vi "UTL_Read_Write Controllers.vi"(8 "error in":errorcluster) -> (0 "error out":errorcluster, 2 "StatusCtrl":T1(array[cluster]), 5 "Results":dbl[][][](array[numeric]))   [LabVIEW 2024]
uses:
  <vilib>/Plasmionique/MB Master/MB_Master_Serial/MB_Master_Serial.lvclass
  Variable global de carga.vi
  <vilib>/Plasmionique/MB Master/MB Master.lvlib
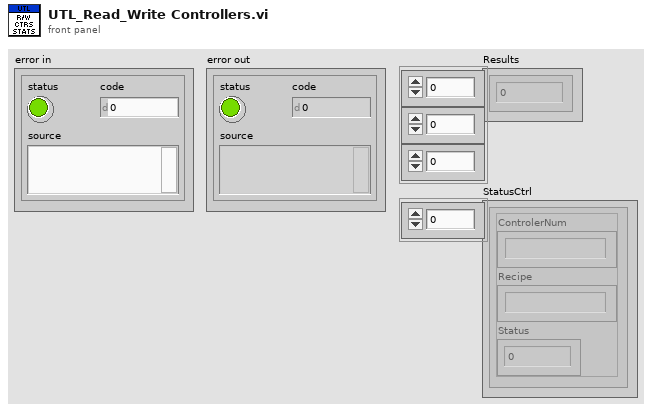
[diagram p1: front panel]
types:
  T1 = cluster{"ControlerNum":string, "Recipe":string, "Status":u32}[]
  T2 = typedef "Control 2.ctl" = refnum<class "MB_Master_Serial.lvclass">[]
  T3 = cluster{"ControlerNum":string, "Recipe":string, "Status":u32}
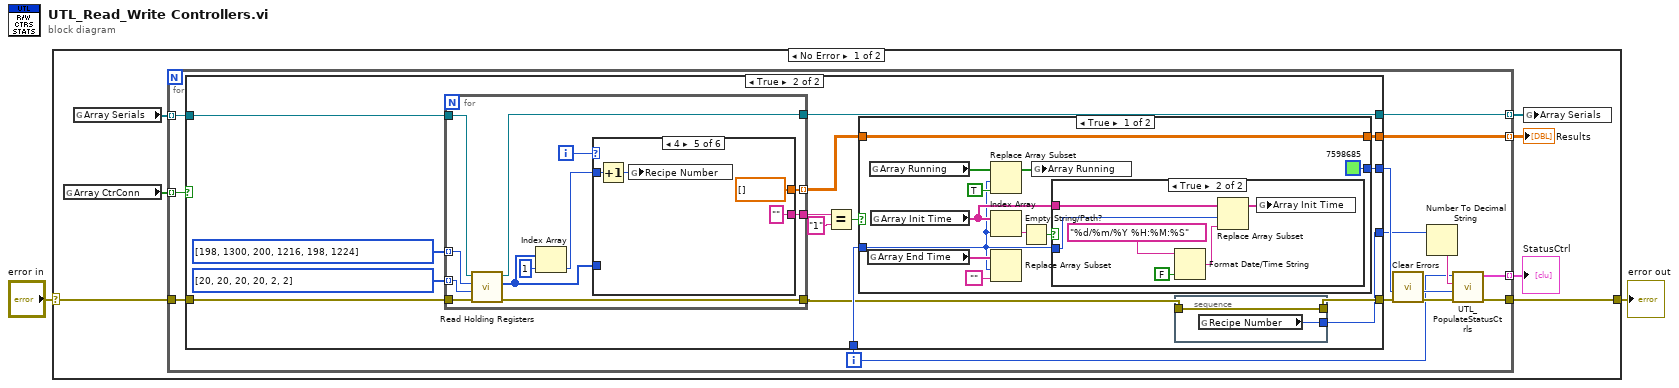
[diagram p0: block diagram]
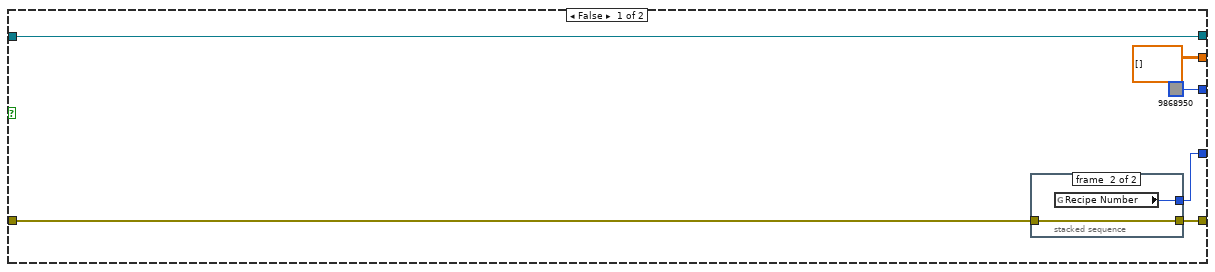
[diagram p2: hidden frame]
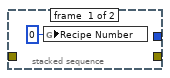
[diagram p3: hidden frame]
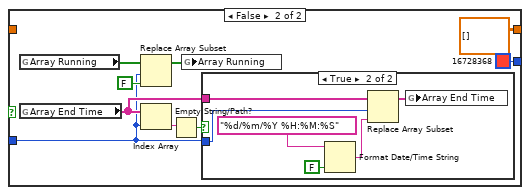
[diagram p5: hidden frame]
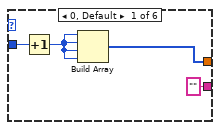
[diagram p7: hidden frame]
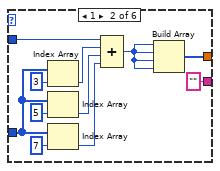
[diagram p8: hidden frame]
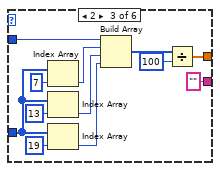
[diagram p9: hidden frame]
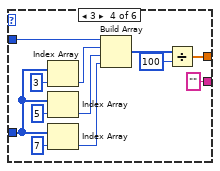
[diagram p10: hidden frame]
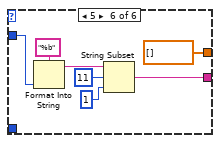
[diagram p11: hidden frame]
diagram:
  n1 = case shown="No Error" "error in" {
    selector: "error in" -> [w8 w143]
    tunnel: [w9 w143] -> w1
    frame No Error {
      n2 = global read "Variable global de carga.vi" "Array CtrConn"() -> (w3:bool[])
      n3 = global read "Variable global de carga.vi" "Array Serials"() -> (w7:T2)
      n4 = for {
        tunnel: w7 -> [w21] mode=indexing
        tunnel: [w20] -> w6 mode=indexing
        tunnel: [w19] -> w5 mode=indexing
        tunnel: w8 -> [w22]
        tunnel: [w18] -> w9
        tunnel: [w17] -> w4 mode=indexing
        tunnel: w3 -> [w11] mode=indexing
        i -> [w12]
        n5 = case shown="True" w11 {
          tunnel: w22 -> [w23 w46]
          tunnel: w21 -> [w28 w41]
          tunnel: [w28 w40] -> w20
          tunnel: [dbl[][] [] w37] -> w19
          tunnel: w12 -> [_ w36]
          tunnel: [w24 w33] -> w14
          tunnel: [u32 9868950 ("Status") w35] -> w13
          tunnel: [w25 w32] -> w10
          frame False {
            n6 = stacked-sequence {
              tunnel: [_ w31] -> w25
              tunnel: [_ w30] -> w24
              tunnel: w23 -> [_ w30]
              frame #0 {
                n7 = global write "Variable global de carga.vi" "Recipe Number"(u16 0 ("Recipe Number")) -> ()
              }
              frame #1 {
                n8 = global read "Variable global de carga.vi" "Recipe Number"() -> (w31:u16)
              }
            }
          }
          frame True {
            n9 = for {
              tunnel: i32[] [198, 1300, 200, 1216, 198, 1224] -> [w88] mode=indexing
              tunnel: [w91] -> w40
              tunnel: [w92] -> w34
              tunnel: [w89] -> w38 mode=indexing
              tunnel: i32[] [20, 20, 20, 20, 2, 2] -> [w87] mode=indexing
              tunnel: w46 -> [w83]
              tunnel: w41 -> [w82]
              tunnel: [w81] -> w42
              i -> [w90]
              n10 = call <vilib>:"Read Holding Registers.vi"("error in (no error)"=w83, "quantity"=w87, "starting address"=w88, "MB session in"=w82) -> ("error out"=w92:errorcluster, "Registers"=w84:u16[], "MB session out"=w91:refnum<class "MB_Master_Serial.lvclass">)  [unwired: 5 in]
              n11 = Index Array(array=w84, index=1) -> (element=w85:u16)
              n12 = case shown="4" w90 {
                tunnel: w84 -> [_ w104 w116 w128 _ _]
                tunnel: [w95 w99 w110 w122 dbl[] [] dbl[] []] -> w89
                tunnel: w85 -> [w94 w98 w109 w121 w135 w138]
                tunnel: ["" "" "" "" "" w136] -> w81
                frame 0, Default {
                  n13 = Increment(x=w94) -> (x+1=w96:u16)
                  n14 = Build Array(w96, w96, w96, w96) -> (w95:u16[])
                }
                frame 1 {
                  n15 = Index Array(array=w104, index=3) -> (element=w103:u16)
                  n16 = Index Array(array=w104, index=5) -> (element=w102:u16)
                  n17 = Index Array(array=w104, index=7) -> (element=w101:u16)
                  n18 = Compound Arithmetic op=ADD(w98, w103, w102, w101) -> (w100:u16)
                  n19 = Build Array(w100, w100, w100, w100) -> (w99:u16[])
                }
                frame 2 {
                  n20 = Index Array(array=w116, index=7) -> (element=w115:u16)
                  n21 = Index Array(array=w116, index=13) -> (element=w114:u16)
                  n22 = Index Array(array=w116, index=19) -> (element=w113:u16)
                  n23 = Build Array(w109, w115, w114, w113) -> (w111:u16[])
                  n24 = Divide(x=w111, y=100) -> (x/y=w110:dbl[])
                }
                frame 3 {
                  n25 = Index Array(array=w128, index=3) -> (element=w127:u16)
                  n26 = Index Array(array=w128, index=5) -> (element=w126:u16)
                  n27 = Index Array(array=w128, index=7) -> (element=w125:u16)
                  n28 = Build Array(w121, w127, w126, w125) -> (w123:u16[])
                  n29 = Divide(x=w123, y=100) -> (x/y=w122:dbl[])
                }
                frame 4 {
                  n30 = Increment(x=w135) -> (x+1=w132:u16)
                  n31 = global write "Variable global de carga.vi" "Recipe Number"(w132) -> ()
                }
                frame 5 {
                  n32 = Format Into String(format string="%b", w138) -> (resulting string=w142:string)  [unwired: 2 in, 1 out]
                  n33 = String Subset(string=w142, offset (0)=11, length (rest)=1 ("length (rest)")) -> (substring=w136:string)
                }
              }
            }
            n34 = Equal?(x=w42, y="1") -> (x = y?=w39:bool)
            n35 = case shown="True" w39 {
              tunnel: w36 -> [w51 w68]
              tunnel: w38 -> [w50 _]
              tunnel: [w50 dbl[][] []] -> w37
              tunnel: [u32 7598685 ("Status 3") u32 16728368 ("Status 4")] -> w35
              frame True {
                n36 = global read "Variable global de carga.vi" "Array End Time"() -> (w53:string[])
                n37 = global read "Variable global de carga.vi" "Array Running"() -> (w55:bool[])
                n38 = global read "Variable global de carga.vi" "Array Init Time"() -> (w57:string[])
                n39 = Replace Array Subset(array=w55, new element=TRUE, index=w51) -> (w54:bool[])
                n40 = Index Array(array=w57, index=w51) -> (element=w59:string)
                n41 = Replace Array Subset(array=w53, new element="" ("new element/subarray"), index=w51) -> ()  [unwired: 1 out]
                n42 = Empty String/Path?(string/path=w59) -> (empty?=w58:bool)
                n43 = global write "Variable global de carga.vi" "Array Running"(w54) -> ()
                n44 = case shown="True" w58 {
                  tunnel: w51 -> [_ w62]
                  tunnel: w57 -> [_ w63]
                  frame False {
                  }
                  frame True {
                    n45 = Format Date/Time String(time format string (%c)="%d/%m/%Y %H:%M:%S", UTC format=FALSE) -> (date/time string=w60:string)  [unwired: 1 in]
                    n46 = Replace Array Subset(array=w63, new element=w60, index=w62) -> (w61:string[])
                    n47 = global write "Variable global de carga.vi" "Array Init Time"(w61) -> ()
                  }
                }
              }
              frame False {
                n48 = global read "Variable global de carga.vi" "Array Running"() -> (w70:bool[])
                n49 = global read "Variable global de carga.vi" "Array End Time"() -> (w72:string[])
                n50 = Replace Array Subset(array=w70, new element=FALSE, index=w68) -> (w69:bool[])
                n51 = Index Array(array=w72, index=w68) -> (element=w74:string)
                n52 = Empty String/Path?(string/path=w74) -> (empty?=w73:bool)
                n53 = global write "Variable global de carga.vi" "Array Running"(w69) -> ()
                n54 = case shown="True" w73 {
                  tunnel: w68 -> [_ w77]
                  tunnel: w72 -> [_ w78]
                  frame False {
                  }
                  frame True {
                    n55 = Format Date/Time String(time format string (%c)="%d/%m/%Y %H:%M:%S", UTC format=FALSE) -> (date/time string=w75:string)  [unwired: 1 in]
                    n56 = Replace Array Subset(array=w78, new element=w75, index=w77) -> (w76:string[])
                    n57 = global write "Variable global de carga.vi" "Array End Time"(w76) -> ()
                  }
                }
              }
            }
            n58 = stacked-sequence {
              tunnel: [w48] -> w32
              tunnel: w34 -> [w47]
              tunnel: [w47] -> w33
              frame #0 {
                n59 = global read "Variable global de carga.vi" "Recipe Number"() -> (w48:u16)
              }
            }
          }
        }
        n60 = call <vilib>:"Clear Errors.vi"("error in (no error)"=w14) -> ("error out"=w15:errorcluster)  [unwired: 5 in, 1 out]
        n61 = Number To Decimal String(number=w10) -> (decimal integer string=w16:string)  [unwired: 1 in]
        n62 = call "UTL_PopulateStatusCtrls.vi"("error in (no error)"=w15, "Status"=w13, "Recipe"=w16, "ComNum"=w12) -> ("error out"=w18:errorcluster, "output cluster"=w17:T3)  [unwired: 6 in]
      }
      "Results" <- w5
      "StatusCtrl" <- w4
      n63 = global write "Variable global de carga.vi" "Array Serials"(w6) -> ()
    }
    frame Error {
    }
  }
  "error out" <- w1
